vi "光学防抖（滑稽）.vi"(11 "布尔输入":bool) -> (3 "布尔输出":bool)   [LabVIEW 2017]
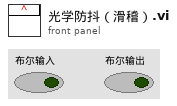
[diagram p1: front panel]
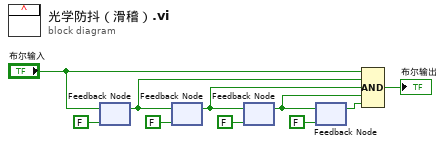
[diagram p0: block diagram]
diagram:
  n1 = feedback #1(FALSE) -> (w8:bool)
  n2 = feedback-in #1("布尔输入") -> ()
  n3 = feedback #2(FALSE) -> (w9:bool)
  n4 = feedback-in #2(w8) -> ()
  n5 = feedback #3(FALSE) -> (w2:bool)
  n6 = feedback-in #3(w9) -> ()
  n7 = feedback #4(FALSE) -> (w1:bool)
  n8 = feedback-in #4(w2) -> ()
  n9 = Compound Arithmetic op=AND ("复合运算")("布尔输入", w8, w9, w2, w1) -> (→"布尔输出":bool)
